vi "CreateParseMessage.vi"(8 "error in (no error)":errorcluster, 11 "Message in":T1) -> (0 "error out":errorcluster, 3 "Message out":T1)   [LabVIEW 2017, in "MessageGen.lvlib"]
uses:
  <vilib>/addons/InsightCM/MessageBus/CodeGen/MessageGen.lvlib
  <vilib>/addons/InsightCM/MessageBus/CodeGen/controls/MessageData.ctl
  <vilib>/addons/InsightCM/MessageBus/CodeGen/controls/MessageType.ctl
  <vilib>/addons/InsightCM/MessageBus/CodeGen/controls/Parameter.ctl
  <vilib>/addons/InsightCM/MessageBus/CodeGen/controls/ParameterType.ctl
  <vilib>/LabVIEW Icon API/API_Text.ctl
  <vilib>/LabVIEW Icon API/LabVIEW Icon API.lvlib
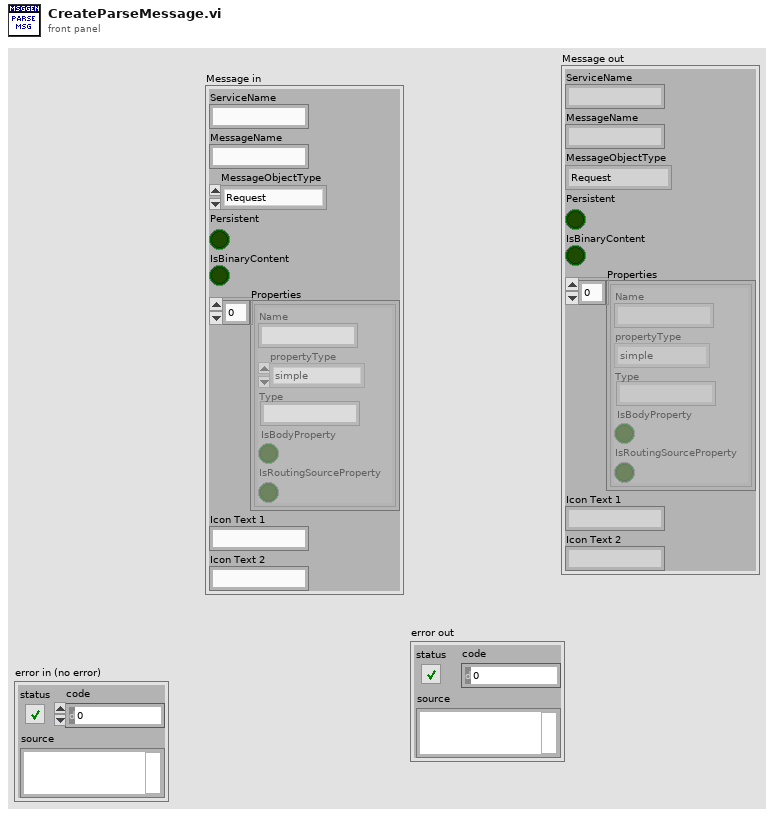
[diagram p1: front panel]
types:
  T1 = typedef "MessageGen.lvlib/MessageData.ctl" = cluster{"ServiceName":string, "MessageName":string, "MessageObjectType":T2, "Persistent":bool, "IsBinaryContent":bool, "Properties":T3[], "Icon Text 1":string, "Icon Text 2":string}
  T2 = typedef "MessageGen.lvlib/MessageType.ctl" = enum16{"Request", "Response", "Broadcast", "RoutedMessage"}
  T3 = typedef "MessageGen.lvlib/Parameter.ctl" = cluster{"Name":string, "propertyType":T4, "Type":string, "IsBodyProperty":bool, "IsRoutingSourceProperty":bool}
  T4 = typedef "MessageGen.lvlib/ParameterType.ctl" = enum16{"simple", "bytearray", "dateTime", "list", "map", "object"}
  T5 = typedef "LabVIEW Icon API.lvlib/API_Text.ctl" = cluster{"Line 1 text":string, "Line 2 text":string, "Line 3 text":string, "Line 4 text":string}
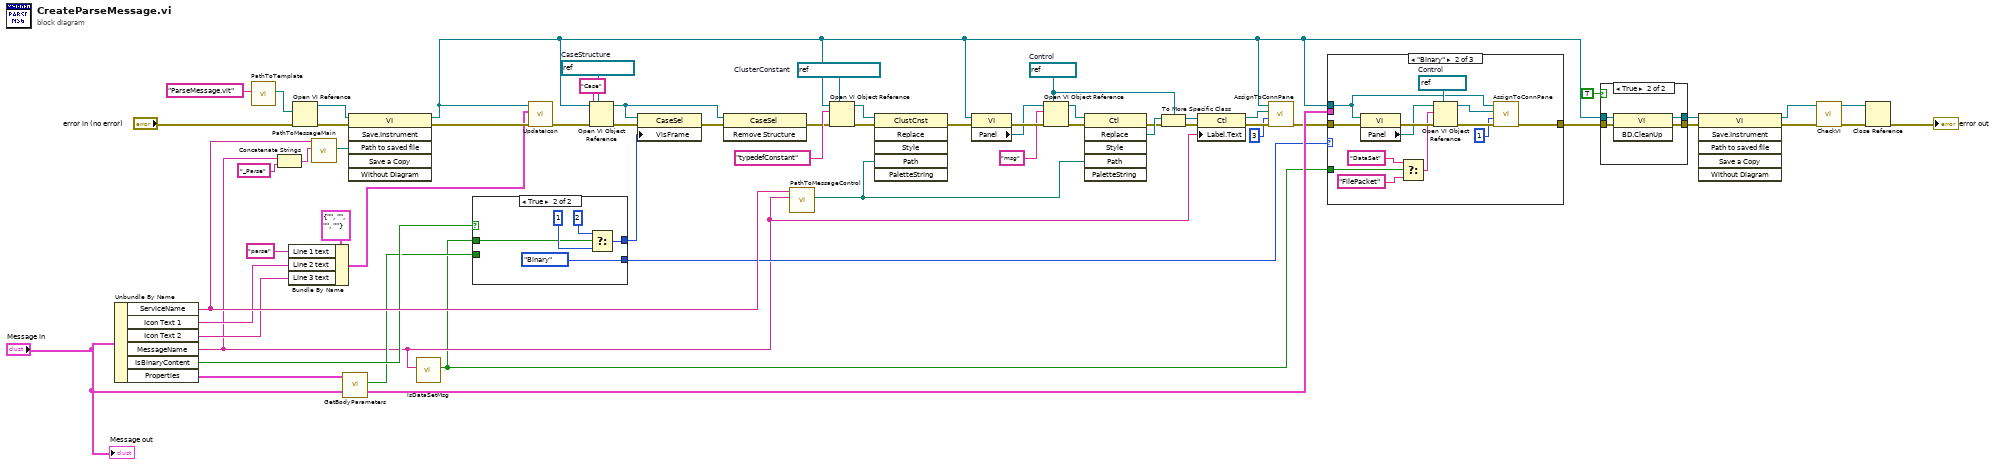
[diagram p0: block diagram]
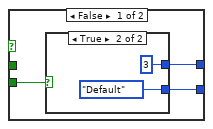
[diagram p2: hidden frame]
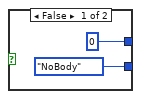
[diagram p3: hidden frame]
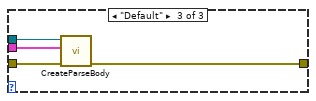
[diagram p6: hidden frame]
diagram:
  w32 = refnum<vi> refnum  # Control
  w36 = refnum<vi> refnum  # ClusterConstant
  w48 = refnum<vi> refnum  # CaseStructure
  n1 = Unbundle By Name("Message in") -> ("ServiceName"=w34:string, "Icon Text 1"=w8:string, "Icon Text 2"=w7:string, "MessageName"=w2:string, "IsBinaryContent"=w14:bool, "Properties"=w41:T3[])
  n2 = call <vilib>:"PathToTemplate.vi"("TemplateName"="ParseMessage.vit") -> ("Path"=w55:path)  [unwired: 10 in]
  n3 = Concatenate Strings(w2, "_Parse" ("string")) -> (w50:string)
  n4 = Bundle By Name(cluster=T5 {"Line 1 text"="", "Line 2 text"="", "Line 3 text"="", "Line 4 text"=""} ("Text"), "Line 1 text"="parse" ("method"), "Line 2 text"=w8, "Line 3 text"=w7) -> (w6:T5)
  n5 = Open VI Reference(vi path=w55, error in (no error)="error in (no error)") -> (vi reference=w57:refnum<vi>, error out=w58:errorcluster)  [unwired: 4 in]
  n6 = call <vilib>:"PathToMessageMain.vi"("VIName"=w50, "Service"=w34) -> ("Path"=w49:path)  [unwired: 9 in]
  n7 = call <vilib>:"GetBodyParameters.vi"("Parameters"=w41) -> ("HasBodyParameters"=w13:bool)  [unwired: 9 in, 1 out]
  n8 = invoke class="VI" method="Save.Instrument"(reference=w57, error in=w58, "Path to saved file"=w49) -> (reference out=w4:refnum<vi>, error out=w43:errorcluster)  [unwired: 3 in, 4 out]
  n9 = call <vilib>:"IsDataSetMsg.vi"("MessageName"=w2) -> ("IsDataSet"=w1:bool)  [unwired: 10 in]
  n10 = case shown="True" w14 {
    tunnel: w13 -> [w63 _]
    tunnel: [w62 enum16{"NoBody", "Binary", "Default"}."Binary"] -> w12
    tunnel: [w61 w70] -> w3
    tunnel: w1 -> [_ w68]
    frame False {
      n11 = case shown="True" w63 {
        tunnel: [enum16{"NoBody", "Binary", "Default"}."NoBody" enum16{"NoBody", "Binary", "Default"}."Default"] -> w62
        tunnel: [u32 0 ("Visible Frame") u32 3 ("Visible Frame")] -> w61
        frame False {
        }
        frame True {
        }
      }
    }
    frame True {
      n12 = Select(t=u32 2 ("Visible Frame"), s=w68, f=u32 1 ("Visible Frame")) -> (s? t:f=w70:u32)
    }
  }
  n13 = call <vilib>:"UpdateIcon.vi"("error in (no error)"=w43, "Text"=w6, "VI Refnum in"=w4) -> ("error out"=w42:errorcluster)  [unwired: 7 in, 1 out]
  n14 = Open VI Object Reference(7:w48, 8:w42, 10:"Case" ("name/order"), 11:w4) -> (0:w44:errorcluster, 3:w45:refnum<vi>)
  n15 = property class="CaseSel"(reference=w45, error in=w44, "VisFrame"=w3) -> (error out=w46:errorcluster)  [unwired: 1 out]
  n16 = invoke class="CaseSel" method="Remove Structure"(reference=w45, error in=w46) -> (error out=w35:errorcluster)  [unwired: 1 in, 2 out]
  n17 = call <vilib>:"PathToMessageControl.vi"("ControlName"=w2, "Service"=w34) -> ("Path"=w22:path)  [unwired: 9 in]
  n18 = Open VI Object Reference(7:w36, 8:w35, 10:"typedefConstant" ("name/order"), 11:w4) -> (0:w37:errorcluster, 3:w38:refnum<vi>)
  n19 = invoke class="ClustCnst" method="Replace"(reference=w38, error in=w37, "Path"=w22) -> (error out=w23:errorcluster)  [unwired: 3 in, 5 out]
  n20 = property class="VI"(reference=w4, error in=w23) -> (error out=w26:errorcluster, "Panel"=w25:refnum<vi>)  [unwired: 1 out]
  n21 = Open VI Object Reference(7:w32, 8:w26, 10:"msg" ("name/order"), 11:w25) -> (0:w28:errorcluster, 3:w27:refnum<vi>)
  n22 = invoke class="Ctl" method="Replace"(reference=w27, error in=w28, "Path"=w22) -> (error out=w29:errorcluster, "Replace"=w31:refnum<vi>)  [unwired: 3 in, 4 out]
  n23 = To More Specific Class(target class=w32, reference=w31, error in=w29) -> (specific class reference=w33:refnum<vi>, error out=w30:errorcluster)
  n24 = property class="Ctl"(reference=w33, error in=w30, "Label.Text"=w2) -> (reference out=w20:refnum<vi>, error out=w21:errorcluster)
  n25 = call <vilib>:"AssignToConnPane.vi"("error in (no error)"=w21, "term index"=u32 3, "Control"=w20, "vi reference"=w4) -> ("error out"=w18:errorcluster)  [unwired: 7 in]
  n26 = case shown="\"Binary\"" w12 {
    tunnel: "Message in" -> [_ _ w90]
    tunnel: [w73 w78 w89] -> w5
    tunnel: w4 -> [_ w79 w88]
    tunnel: w18 -> [w73 w80 w87]
    tunnel: w1 -> [_ w77 _]
    frame "NoBody" {
    }
    frame "Binary" {
      w84 = refnum<vi> refnum  # Control
      n27 = property class="VI"(reference=w79, error in=w80) -> (error out=w83:errorcluster, "Panel"=w82:refnum<vi>)  [unwired: 1 out]
      n28 = Select(t="DataSet" ("name/order"), s=w77, f="FilePacket" ("name/order")) -> (s? t:f=w74:string)
      n29 = Open VI Object Reference(7:w84, 8:w83, 10:w74, 11:w82) -> (0:w85:errorcluster, 3:w86:refnum<vi>)
      n30 = call <vilib>:"AssignToConnPane.vi"("error in (no error)"=w85, "term index"=u32 1, "Control"=w86, "vi reference"=w79) -> ("error out"=w78:errorcluster)  [unwired: 7 in]
    }
    frame "Default" {
      n31 = call <vilib>:"CreateParseBody.vi"("error in (no error)"=w87, "Message in"=w90, "VI reference"=w88) -> ("error out"=w89:errorcluster)  [unwired: 8 in]
    }
  }
  n32 = case shown="True" TRUE {
    tunnel: w5 -> [w91 w96]
    tunnel: [w91 w95] -> w17
    tunnel: w4 -> [w92 w94]
    tunnel: [w92 w93] -> w16
    frame False {
    }
    frame True {
      n33 = invoke class="VI" method="BD.CleanUp"(reference=w94, error in=w96) -> (reference out=w93:refnum<vi>, error out=w95:errorcluster)  [unwired: 1 in, 1 out]
    }
  }
  n34 = invoke class="VI" method="Save.Instrument"(reference=w16, error in=w17) -> (reference out=w54:refnum<vi>, error out=w52:errorcluster)  [unwired: 4 in, 4 out]
  n35 = call <vilib>:"CheckVI.vi"("error in (no error)"=w52, "VI ref"=w54) -> ("error out"=w51:errorcluster, "VI ref out"=w53:refnum<vi>)  [unwired: 8 in]
  n36 = Close Reference(reference=w53, error in (no error)=w51) -> (error out=→"error out":errorcluster)
  "Message out" <- "Message in"
